vi "ToggleByRoomName.vi"(0 "reference in":refnum<class "SecuritySystem.lvclass">, 2 "RoomName":string, 5 "Error In":errorcluster) -> (14 "reference out":refnum<class "SecuritySystem.lvclass">, 19 "Error Out":errorcluster)   [LabVIEW 2024, in "SecuritySystem.lvclass"]
uses:
  SecuritySystem.lvclass
  House/Room_class/Room.lvclass
  SecuritySystem.lvclass/SecuritySystem.ctl
  Devices/Security_class/Security.lvclass
panel:
  # "Connector Pane"
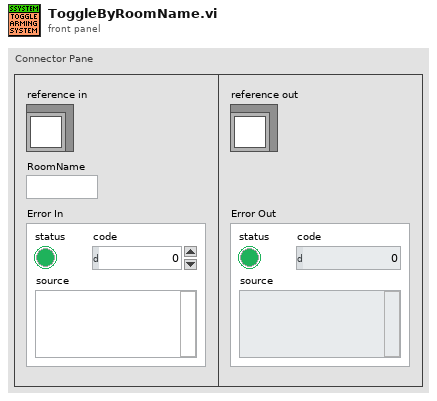
[diagram p1: front panel]
types:
  T1 = typedef "SecuritySystem.lvclass/ObjectAttributes.ctl" = cluster{"Rooms":T2}
  T2 = typedef "Rooms Map.ctl" = map{string, refnum<class "Room.lvclass">}
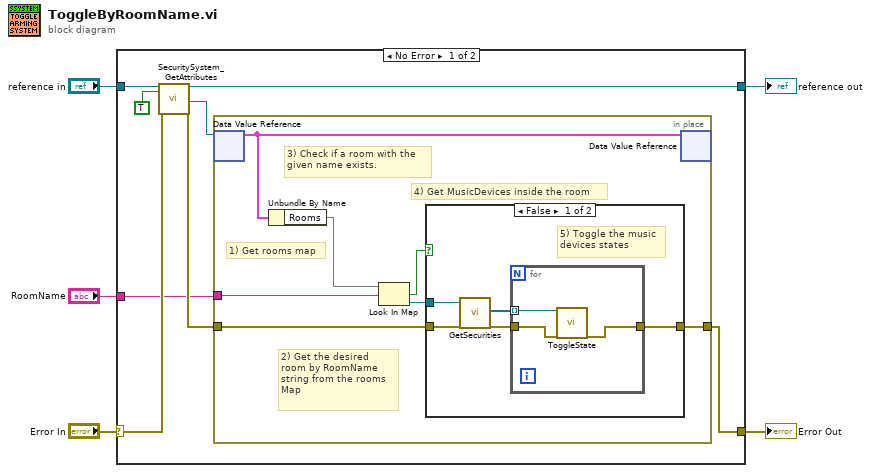
[diagram p0: block diagram]
diagram:
  n1 = case shown="No Error" "Error In" {
    selector: "Error In" -> [w12 w31]
    tunnel: [w7 w31] -> w4
    tunnel: [w11 w30] -> w2
    tunnel: "reference in" -> [w13 w30]
    tunnel: "RoomName" -> [w6 _]
    frame No Error {
      n2 = call "SecuritySystem_GetAttributes.vi"("reference in"=w13, "OnlyGetDvrReference(False)"=TRUE, "Error In"=w12) -> ("reference out"=w11:refnum<class "SecuritySystem.lvclass">, "DataRef"=w9:refnum<data-value>, "Error Out"=w8:errorcluster)  [unwired: 13 in, 1 out]
      n3 = in-place {
        in-place-border: w6 -> [w16]
        in-place-border: w8 -> [w15]
        in-place-border: [w14] -> w7
        # "4) Get MusicDevices inside the room"
        # "3) Check if a room with the\ngiven name exists."
        # "2) Get the desired\nroom by RoomName\nstring from the rooms\nMap"
        # "1) Get rooms map"
        n4 = in-place-dvr #1(w9) -> (w20:T1)  [unwired: 1 out]
        n5 = Unbundle By Name(w20) -> ("Rooms"=w17:T2)
        n6 = Look In Map(map=w17, key=w16) -> (key not found?=w19:bool, value=w18:refnum<class "Room.lvclass">)  [unwired: 1 in]
        n7 = case shown="False" w19 {
          tunnel: w18 -> [w25 _]
          tunnel: w15 -> [w22 w29]
          tunnel: [w21 w29] -> w14
          frame False {
            # "5) Toggle the music\ndevices states"
            n8 = call-dynamic "GetSecurities.vi"("reference in"=w25, "Error In"=w22) -> ("Securities"=w24:refnum<class "Security.lvclass">[], "Error Out"=w23:errorcluster)  [unwired: 15 in, 1 out]
            n9 = for {
              tunnel: w24 -> [w26] mode=indexing
              tunnel: w23 -> [w28]
              tunnel: [w27] -> w21
              n10 = call "ToggleState.vi"("reference in"=w26, "Error In"=w28) -> ("Error Out"=w27:errorcluster)  [unwired: 16 in, 1 out]
            }
          }
          frame True {
          }
        }
        n11 = in-place-dvr #1(w20) -> ()  [unwired: 2 out]
      }
    }
    frame Error {
    }
  }
  "Error Out" <- w4
  "reference out" <- w2
